vi "Disable Logger by Name.vi"(8 "error in (no error)":errorcluster, 11 "name":string) -> (0 "error out":errorcluster)   [LabVIEW 2018, in "GLog.lvlib"]
uses:
  GLog.lvlib
  registry/Registry.lvlib
panel:
  # "Connector Pane"
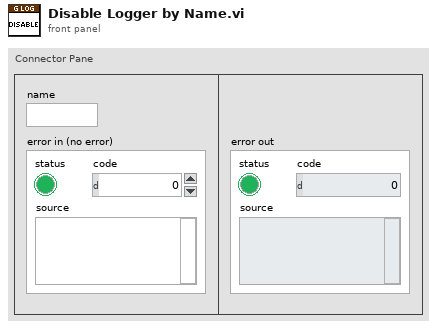
[diagram p1: front panel]
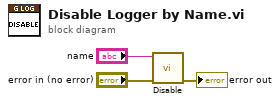
[diagram p0: block diagram]
diagram:
  n1 = call "Disable.vi"("error in (no error)"="error in (no error)", "logger name"="name") -> ("error out"=→"error out":errorcluster)  [unwired: 9 in]
